vi "Apply Optical PWM To Voltage.vi"(0 "Pulse Train in":refnum<class "Pulse Train.lvclass">, 5 "Level in":refnum<class "Level.lvclass">, 9 "Min voltage":dbl, 11 "error in (no error)":errorcluster) -> (4 "Pulse Train out":refnum<class "Pulse Train.lvclass">, 6 "Level out":refnum<class "Level.lvclass">, 8 "Pulse width (us)":dbl, 10 "PWM factor":dbl, 15 "error out":errorcluster)   [LabVIEW 2015, in "Pulse Train.lvclass"]
uses:
  Pulse Train.lvclass
  Level/Level.lvclass
  Utility VIs/Math VIs/dB to Linear (scalar).vi
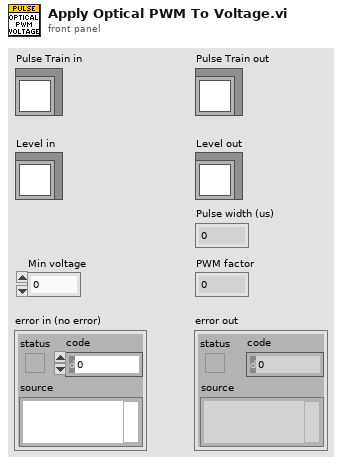
[diagram p1: front panel]
types:
  T1 = typedef "Level.lvclass/LevelUnits.ctl" = enum16{"dB atten", "dB SPL", "dB Vrms", "Volts", "dB mW", "mW", "dB HL", "dB SL"}
  T2 = cluster{"Volts":dbl[], "Width":dbl[], "Rate":dbl[], "Power":dbl[][][][]}
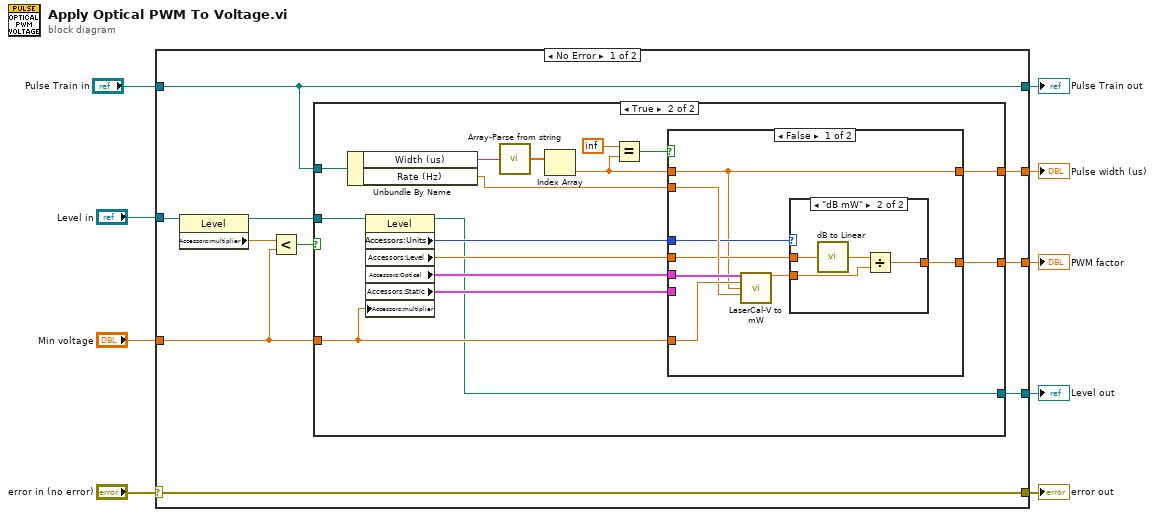
[diagram p0: block diagram]
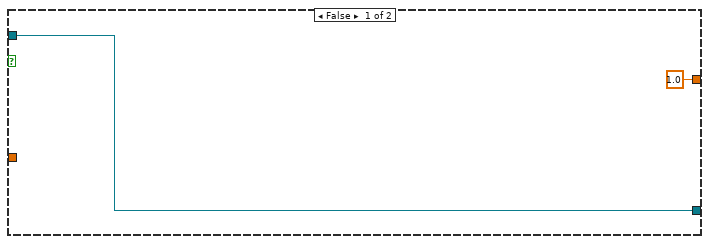
[diagram p2: hidden frame]
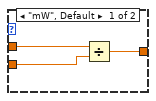
[diagram p3: hidden frame]
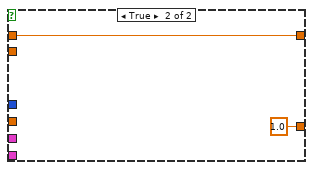
[diagram p4: hidden frame]
diagram:
  n1 = case shown="No Error" "error in (no error)" {
    selector: "error in (no error)" -> [w19 w57]
    tunnel: [w19 w57] -> w8
    tunnel: [w11 w56] -> w6
    tunnel: "Pulse Train in" -> [w11 w56]
    tunnel: "Level in" -> [w18 w55]
    tunnel: "Min voltage" -> [w14 _]
    tunnel: [w13 w55] -> w3
    tunnel: [w12 _] -> w2
    tunnel: [w10 _] -> w1
    frame No Error {
      n2 = property class="Level"(reference=w18) -> (reference out=w16:refnum<class "Level.lvclass">, "Accessors:multiplier"=w17:dbl)  [unwired: 1 in, 1 out]
      n3 = Less?(x=w17, y=w14) -> (x < y?=w15:bool)
      n4 = case shown="True" w15 {
        tunnel: w16 -> [w21 w35]
        tunnel: w11 -> [_ w23]
        tunnel: w14 -> [_ w28]
        tunnel: [w21 w25] -> w13
        tunnel: [1.0 w24] -> w12
        tunnel: [_ w22] -> w10
        frame False {
        }
        frame True {
          n5 = Unbundle By Name(w23) -> ("Width (us)"=w36:string, "Rate (Hz)"=w31:dbl)
          n6 = property class="Level"(reference=w35, "Accessors:multiplier"=w28) -> (reference out=w25:refnum<class "Level.lvclass">, "Accessors:Units"=w27:T1, "Accessors:Level"=w26:dbl, "Accessors:Optical"=w30:T2, "Accessors:Static"=w29:cluster{"Voltage":dbl[], "Power":dbl[]})  [unwired: 1 in, 1 out]
          n7 = call "Array-Parse from string.vi"("String"=w36) -> ("Array"=w37:dbl[])  [unwired: 13 in, 1 out]
          n8 = Index Array(array=w37) -> (element=w32:dbl)  [unwired: 1 in]
          n9 = Equal?(x=inf, y=w32) -> (x = y?=w33:bool)
          n10 = case shown="False" w33 {
            tunnel: w32 -> [w38 w53]
            tunnel: w31 -> [w43 _]
            tunnel: w30 -> [w45 _]
            tunnel: w29 -> [_ _]
            tunnel: w28 -> [w44 _]
            tunnel: w27 -> [w42 _]
            tunnel: w26 -> [w40 _]
            tunnel: [w39 1.0] -> w24
            tunnel: [w38 w53] -> w22
            frame False {
              n11 = call "LaserCal-V to mW.vi"("I-O"=w45, "Volts"=w44, "Pulse width (us)"=w38, "Pulse rate (Hz)"=w43) -> ("Power (mW)"=w41:dbl)  [unwired: 10 in, 1 out]
              n12 = case shown="\"dB mW\"" w42 {
                tunnel: w41 -> [w47 w51]
                tunnel: w40 -> [w48 w52]
                tunnel: [w46 w50] -> w39
                frame "mW", Default {
                  n13 = Divide(x=w48, y=w47) -> (x/y=w46:dbl)
                }
                frame "dB mW" {
                  n14 = call-poly "dB to Linear.vi"("dB"=w52) -> ("linear"=w49:dbl)
                  n15 = Divide(x=w49, y=w51) -> (x/y=w50:dbl)
                }
              }
            }
            frame True {
            }
          }
        }
      }
    }
    frame Error {
    }
  }
  "error out" <- w8
  "Pulse Train out" <- w6
  "Level out" <- w3
  "PWM factor" <- w2
  "Pulse width (us)" <- w1
